vi "Rec_calculate Z_2.vi"(4 "Error":dbl[][](array[numeric]), 6 "拟合半径":i32=2, 7 "info":T3={"data name"="", "ROI ref"=refnum, "cali ref"=refnum, "参考球？"=FALSE, "LUT"=[], "Cali array"=[], "修正次数"=2, "R_step"=0.4, "sample(quar)"=12}, 9 "xy array":cluster{"X Centroid":sgl, "Y Centroid":sgl}[](array[cluster]), 10 "tracking":T1 {"centroid"."Y Centroid" format="%.2f"; "centroid"."X Centroid" format="%.2f"; "ROI Des out"."Contours"."Type" items=["No Selection", "Point", "Line", "Rectangle", "Oval", "Polygon", "Freehand Region", "Annulus", "Unused2", "Unused3", "Broken Line", "Freehand Line", "Rotated Rectangle"]}, 11 "帧数":i32) -> (2 "tracking Out":T1 {"centroid"."Y Centroid" format="%.2f"; "centroid"."X Centroid" format="%.2f"; "ROI Des out"."Contours"."Type" items=["No Selection", "Point", "Line", "Rectangle", "Oval", "Polygon", "Freehand Region", "Annulus", "Unused2", "Unused3", "Broken Line", "Freehand Line", "Rotated Rectangle"]}, 3 "Dif LUT":cluster{"LUT":dbl[], dbl[]}(graph))   [LabVIEW 2017]
uses:
  <vilib>/Analysis/NI_AALPro.lvlib
  <vilib>/vision/Image Controls.llb/IMAQ Image.ctl
  control/bead info.ctl
  control/Bead track.ctl
panel:
  out "radial profile array":dbl[][](array[numeric])
  out "xyz value":dbl[][](array[numeric])
  out "min LUT":cluster{dbl[], "Best Polynomial Fit":dbl[]}(graph)
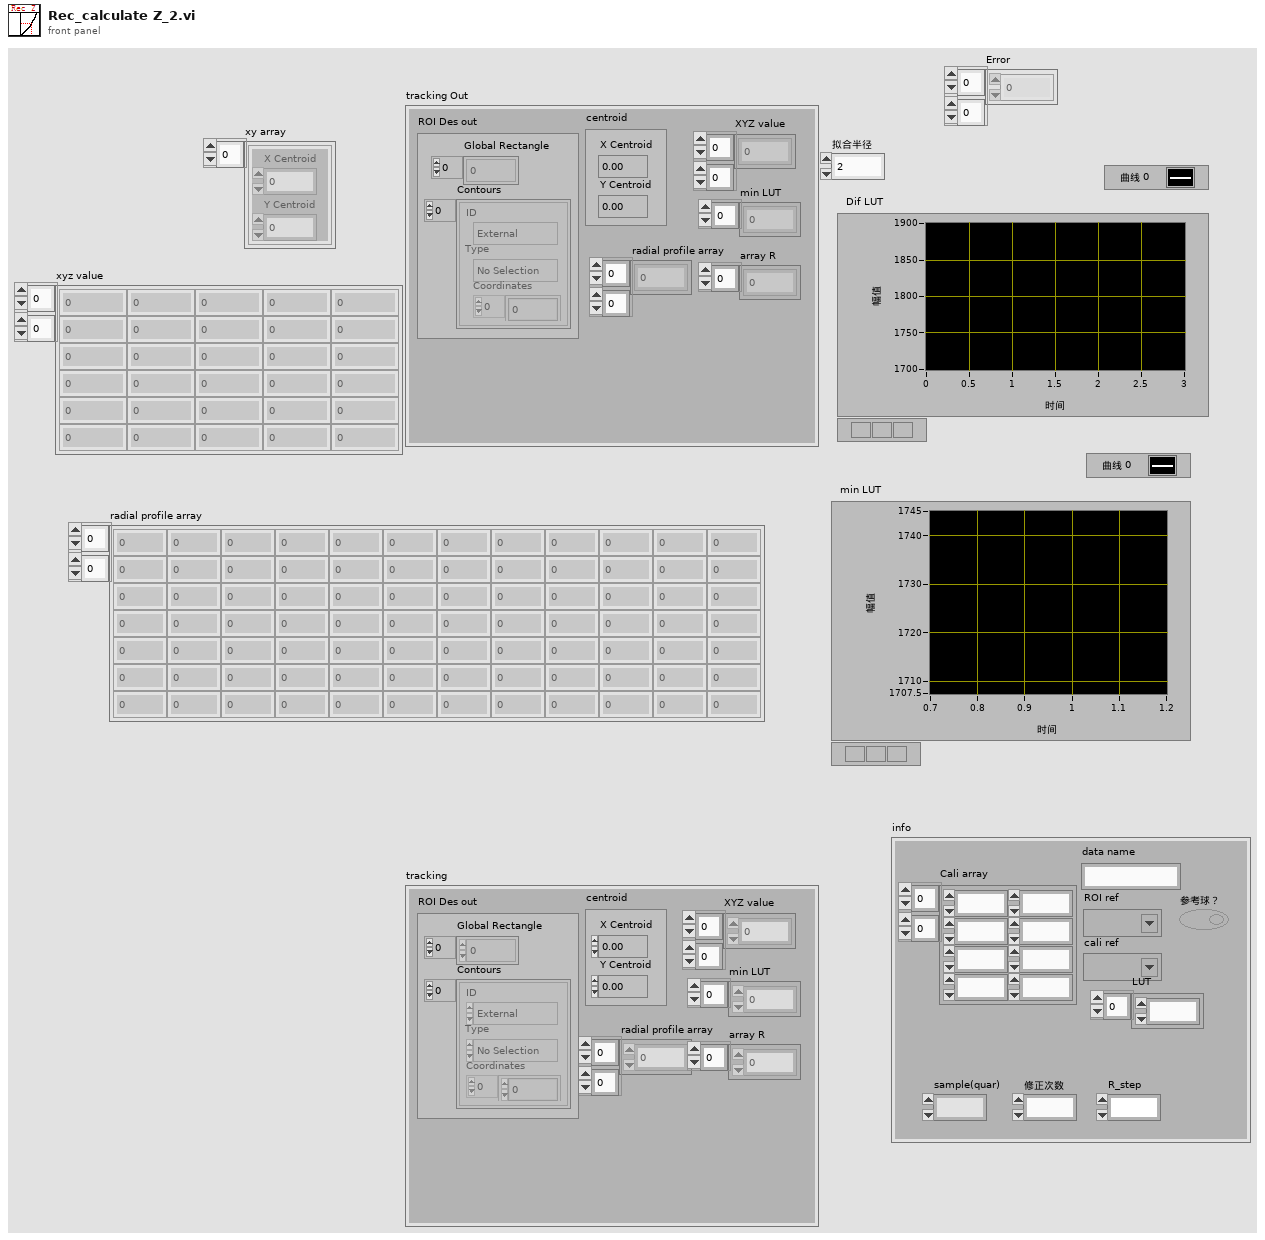
[diagram p1: front panel]
types:
  T1 = typedef "Bead track.ctl" = cluster{"XYZ value":dbl[][], "radial profile array":dbl[][], "min LUT":dbl[], "ROI Des out":T2, "array R":dbl[], "centroid":cluster{"X Centroid":sgl, "Y Centroid":sgl}}
  T2 = typedef "ROI Descriptor" = cluster{"Global Rectangle":i32[], "Contours":cluster{"ID":enum32{"External", "Internal"}, "Type":u32, "Coordinates":i32[]}[]}
  T3 = typedef "bead info.ctl" = cluster{"data name":string, "ROI ref":T4, "cali ref":T4, "参考球？":bool, "LUT":dbl[], "Cali array":dbl[][], "修正次数":i32, "R_step":dbl, "sample(quar)":i32}
  T4 = typedef "IMAQ Image.ctl" = refnum<image>
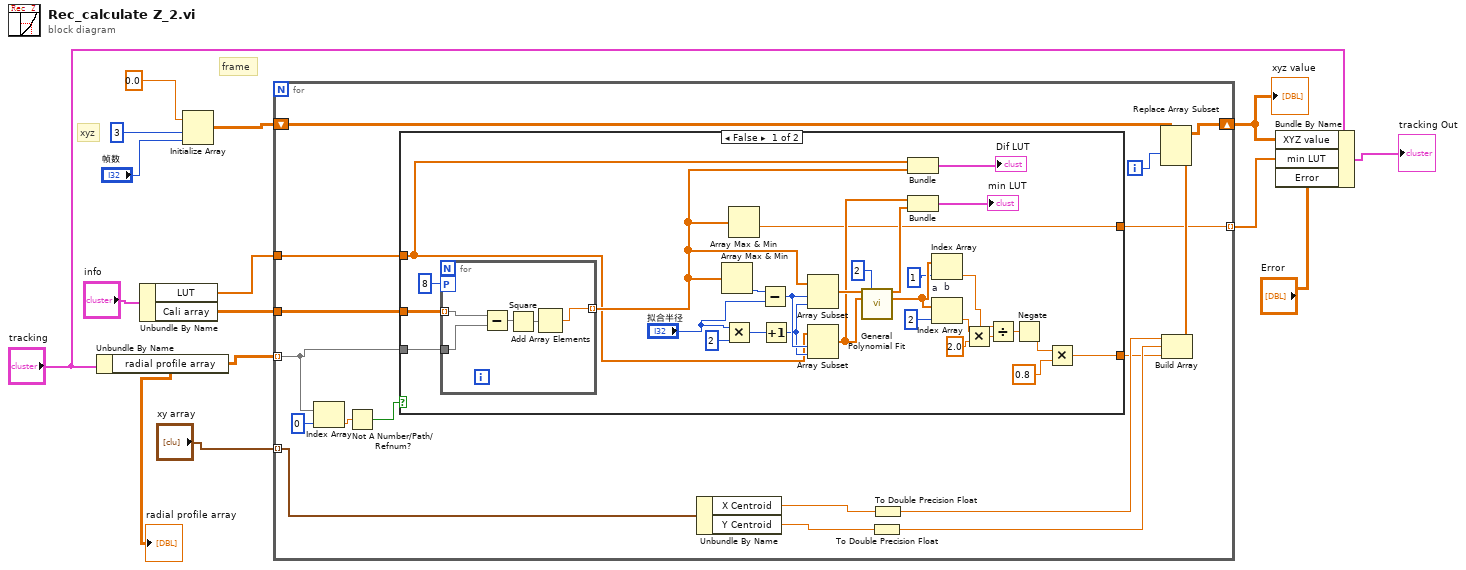
[diagram p0: block diagram]
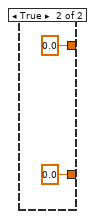
[diagram p2: hidden frame]
diagram:
  # "frame"
  # "xyz"
  n1 = Unbundle By Name("tracking") -> ("radial profile array"=w4:dbl[][])
  "radial profile array" <- w4
  n2 = Unbundle By Name("info") -> ("LUT"=w7:dbl[], "Cali array"=w6:dbl[][])
  n3 = Initialize Array(0.0 ("元素"), 3 ("维数大小"), "帧数") -> (w14:dbl[][])
  n4 = for "For循环" {
    tunnel: w4 -> [w18] mode=indexing
    shift-right: [w23] -> w10
    shift-left: w14 -> [w26]
    tunnel: "xy array" -> [w24] mode=indexing
    tunnel: [w22] -> w9 mode=indexing
    tunnel: w7 -> [w21]
    tunnel: w6 -> [w20]
    i -> [w19]
    n5 = Index Array(array=w18, index=0 ("索引")) -> (element=w16:dbl)
    n6 = Not A Number/Path/Refnum?(number/path/refnum=w16) -> (NaN/Path/Refnum?=w15:bool)
    n7 = case shown="False" w15 {
      tunnel: [w37 0.0] -> w27
      tunnel: [w35 0.0] -> w22
      tunnel: w21 -> [w34 _]
      tunnel: w20 -> [w33 _]
      tunnel: w18 -> [w32 _]
      frame False {
        n8 = for "For循环" {
          tunnel: w32 -> [w65]
          tunnel: [w62] -> w36 mode=indexing
          workers-P: 8 -> [_]
          tunnel: w33 -> [w61] mode=indexing
          n9 = Subtract(x=w61, y=w65) -> (x-y=w64:dbl[])
          n10 = Square(x=w64) -> (x^2=w63:dbl[])
          n11 = Add Array Elements(numeric array=w63) -> (sum=w62:dbl)
        }
        n12 = Array Max & Min(array=w36) -> (min index (indices)=w46:i32)  [unwired: 3 out]
        n13 = Multiply(x="拟合半径", y=2 ("x")) -> (x*y=w50:i32)
        n14 = Array Max & Min(array=w36) -> (min value=w35:dbl)  [unwired: 3 out]
        n15 = Subtract(x=w46, y="拟合半径") -> (x-y=w48:i32)
        n16 = Increment(x=w50) -> (x+1=w47:i32)
        n17 = Array Subset(array=w36, index=w48, length=w47) -> (w45:dbl[])
        n18 = Array Subset(array=w34, index=w48, length=w47) -> (w42:dbl[])
        n19 = call <vilib>:"General Polynomial Fit.vi"("Y"=w45, "polynomial order"=2, "X"=w42) -> ("Best Polynomial Fit"=w43:dbl[], "Polynomial Coefficients"=w58:dbl[])  [unwired: 9 in, 2 out]
        n20 = Bundle("LUT"=w34, w36) -> (→"Dif LUT":cluster{"LUT":dbl[], dbl[]})  [unwired: 1 in]
        n21 = Bundle(w42, "Best Polynomial Fit"=w43) -> (→"min LUT":cluster{dbl[], "Best Polynomial Fit":dbl[]})  [unwired: 1 in]
        n22 = Index Array "b"(array=w58, index=1 ("索引")) -> (element=w54:dbl)
        n23 = Index Array "a"(array=w58, index=2 ("索引")) -> (element=w56:dbl)
        n24 = Multiply(x=w56, y=2.0) -> (x*y=w53:dbl)
        n25 = Divide(x=w54, y=w53) -> (x/y=w52:dbl)
        n26 = Negate(x=w52) -> (-x=w39:dbl)
        n27 = Multiply(x=w39, y=0.8) -> (x*y=w37:dbl)
      }
      frame True {
      }
    }
    n28 = Unbundle By Name(w24) -> ("X Centroid"=w31:sgl, "Y Centroid"=w30:sgl)
    n29 = To Double Precision Float(number=w30) -> (double precision float=w28:dbl)
    n30 = To Double Precision Float(number=w31) -> (double precision float=w29:dbl)
    n31 = Build Array(w29, w28, w27) -> (w25:dbl[])
    n32 = Replace Array Subset(array=w26, new element=w25, index (col)=w19) -> (w23:dbl[][])  [unwired: 1 in]
  }
  "xyz value" <- w10
  n33 = Bundle By Name(cluster="tracking", "XYZ value"=w10, "min LUT"=w9, "Error"="Error") -> (→"tracking Out":T1)
